vi "Perform Active DUT Audio Call Action.vi"(8 "error in (no error)":errorcluster, 9 "Action (Reject)":i32(ring) items=["Reject", "Disconnect", "Accept", "Connect"], 10 "SIM Slot (1)":i32=1, 11 "VISA resource name":refnum<visa-resource-name>) -> (0 "error out":errorcluster, 3 "VISA resource name out":refnum<visa-resource-name>)   [LabVIEW 2020, in "Rohde&Schwarz CMXP Base.lvlib"]
doc: "Controls the audio call connection.\n\nAttributes:\nRSCMXPBASE_ATTR_SELECT_ACTIVE_DUT_SIM_SLOT\nRSCMXPBASE_ATTR_ACTIVE_DUT_AUDIO_CALL_PERFORM_ACTION\n\nRemote-control command:\nPROCedure:DUT:MODem<ModemIdx>:CONTrol:CALL:AUDio"
uses:
  <instrlib>/Rohde&Schwarz CMXP Base/Rohde&Schwarz CMXP Base.lvlib
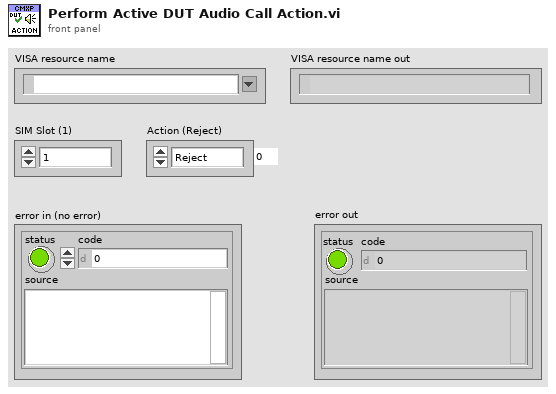
[diagram p1: front panel]
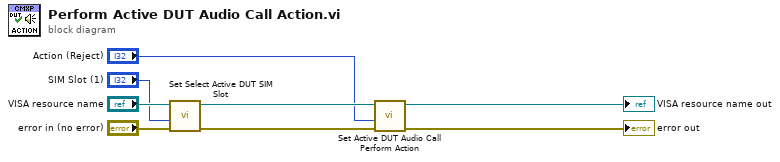
[diagram p0: block diagram]
diagram:
  n1 = call "Set Select Active DUT SIM Slot"("error in (no error)"="error in (no error)", "Select Active DUT SIM Slot (0)"="SIM Slot (1)", "instrument handle"="VISA resource name") -> ("error out"=w3:errorcluster, "instrument handle out"=w4:refnum<visa-resource-name>)  [unwired: 7 in]
  n2 = call "Set Active DUT Audio Call Perform Action"("error in (no error)"=w3, "Active DUT Audio Call Perform Action (0 - Reject)"="Action (Reject)", "instrument handle"=w4) -> ("error out"=→"error out":errorcluster, "instrument handle out"=→"VISA resource name out":refnum<visa-resource-name>)  [unwired: 7 in]
